vi "GetCount.vi"(8 "error in (no error)":errorcluster, 11 "CollectionByRef in":refnum<class "CollectionByRef.lvclass">) -> (0 "error out":errorcluster, 2 "Count":i32, 3 "CollectionByRef out":refnum<class "CollectionByRef.lvclass">)   [LabVIEW 2021, in "Collection.lvlib" / "CollectionByRef.lvclass"]
uses:
  CollectionByRef.lvclass
  CollectionByRef.lvclass/CollectionByRef.ctl
  CollectionByValue/CollectionByValue.lvclass
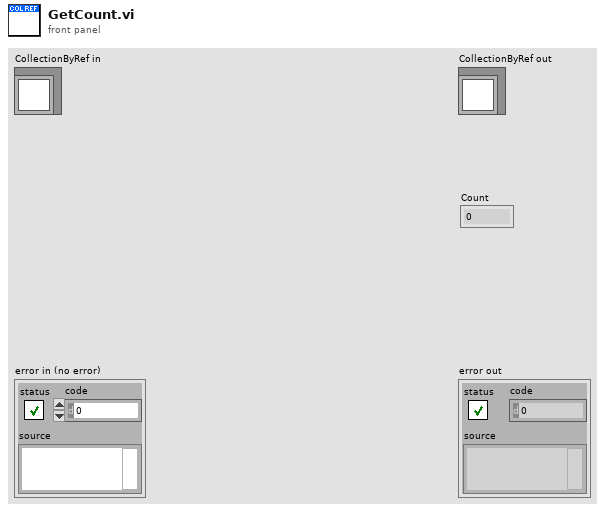
[diagram p1: front panel]
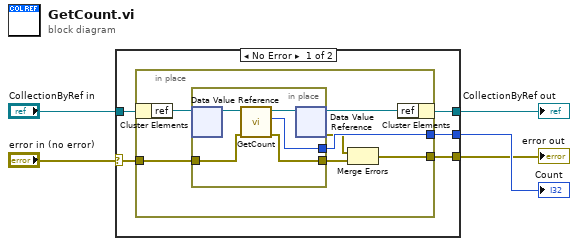
[diagram p0: block diagram]
diagram:
  n1 = case shown="No Error" "error in (no error)" {
    selector: "error in (no error)" -> [w7 w24]
    tunnel: [w9 w23] -> w3
    tunnel: "CollectionByRef in" -> [w10 w23]
    tunnel: [w8 _] -> w2
    tunnel: [w6 w24] -> w1
    frame No Error {
      n2 = in-place {
        in-place-border: [w15] -> w8
        in-place-border: w7 -> [w14]
        in-place-border: [w11] -> w6
        n3 = in-place-cluster #1(w10) -> ("ref"=w17:refnum<data-value>)
        n4 = in-place {
          in-place-border: [w21] -> w15
          in-place-border: w14 -> [w19]
          in-place-border: [w18] -> w12
          n5 = in-place-dvr #2(w17) -> (w22:refnum<class "CollectionByValue.lvclass">)  [unwired: 1 out]
          n6 = call "GetCount.vi"("error in (no error)"=w19, "Collection in"=w22) -> ("error out"=w18:errorcluster, "Count"=w21:i32, "Collection out"=w20:refnum<class "CollectionByValue.lvclass">)  [unwired: 7 in]
          n7 = in-place-dvr #2(w20) -> (w16:refnum<data-value>, w13:errorcluster)
        }
        n8 = Merge Errors(w13, w12) -> (w11:errorcluster)
        n9 = in-place-cluster #1("ref"=w16) -> (w9:refnum<class "CollectionByRef.lvclass">)
      }
    }
    frame Error {
    }
  }
  "error out" <- w1
  "CollectionByRef out" <- w3
  "Count" <- w2
